vi "RequestAndResponseData.vi"(7 "Delay Time (s)":dbl format="%#_13g", 8 "error in (no error)":errorcluster caption="错误输入（无错误）", 9 "sendbuf":string, 10 "conn_num 0":i32, 11 "comm_type  intenettype 1":i32) -> (0 "error out":errorcluster caption="错误输出", 2 "recvbuf out":string, 3 "function return":i32)   [LabVIEW 2015]
uses:
  <userlib>/DMT/DMT.lvlib
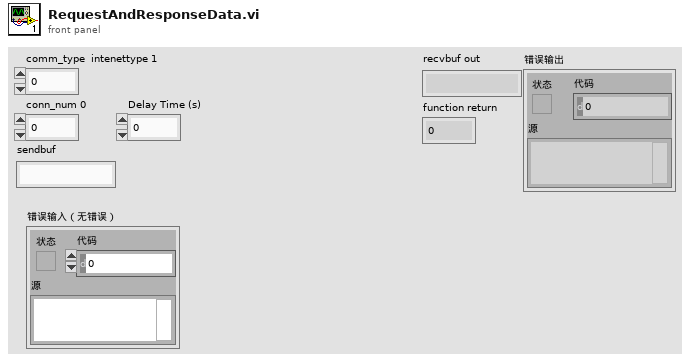
[diagram p1: front panel]
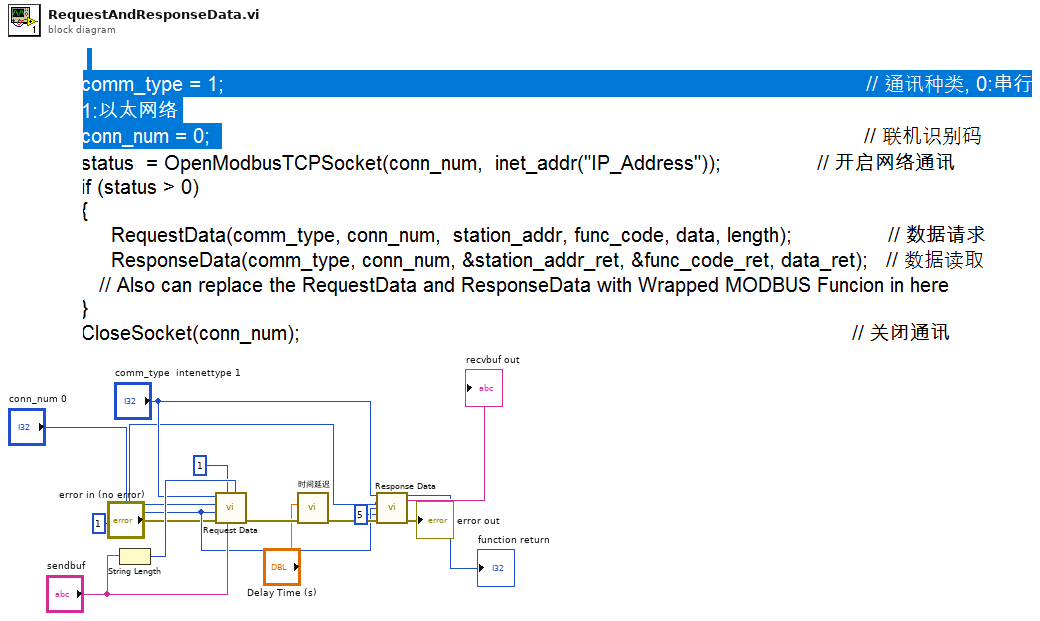
[diagram p0: block diagram]
diagram:
  w7 = 1 ("slave_addr")
  n1 = String Length(string="sendbuf") -> (length=w13:i32)
  n2 = call <userlib>:"Request Data.vi"("sendlen"=w13, "sendbuf"="sendbuf", "func_code"=1, "error in (no error)"="error in (no error)", "slave_addr"=w7, "conn_num"="conn_num 0", "comm_type"="comm_type  intenettype 1") -> ("error out"=w11:errorcluster)  [unwired: 3 in, 1 out]
  n3 = call "时间延迟"("error in (no error)"=w11, "Delay Time (s)"="Delay Time (s)") -> ("error out"=w10:errorcluster)  [unwired: 9 in]
  n4 = call <userlib>:"Response Data.vi"("comm_type"="comm_type  intenettype 1", "conn_num"="conn_num 0", "slave_addr"=w7, "func_code"=5, "error in (no error)"=w10) -> ("recvbuf out"=→"recvbuf out":string, "function return"=→"function return":i32, "error out"=→"error out":errorcluster)  [unwired: 6 in, 2 out]
